vi "Voltage Measurement.vi"() -> ()   [LabVIEW 2021, in "Main.lvlib"]
uses:
  Main.lvlib
  SMU/SMU.lvlib
  DMM/DMM.lvlib
  <instrlib>/niDMM/nidmm.llb/niDMM Resolution in Digits.ctl
  controls/Voltage Config.ctl
  controls/Current Config.ctl
panel:
  out "Current Measurement":dbl
  out "Voltage Measurement":dbl
  in  "Current Config":T1={"Current Limit"=0.01, "Current Limit Range"=0.01} {"Current Limit Range" format="%.3p"; "Current Limit" format="%.3p"}
  in  "Voltage Config":T2={"Voltage Level"=2.0, "Voltage Level Range"=6.0} {"Voltage Level Range" format="%.5p"; "Voltage Level" format="%.5p"}
  out "Signal Out of Range":bool
  out "Measurement":dbl format="%.6p"
  in  "Resolution in Digits":T3=5.5 items=["3 1/2"=3.5, "4 1/2"=4.5, "5 1/2"=5.5, "6 1/2"=6.5, "7 1/2"=7.5]
  in  "Range":dbl=10.0 format="%.2f"
  in  "Device Name":refnum<k15>="Dev1"
  out "error out":errorcluster
  in  "error in":errorcluster
  in  "Vin SMU Channel":string="0"
  in  "Vin SMU":refnum<k15>="Dev1"
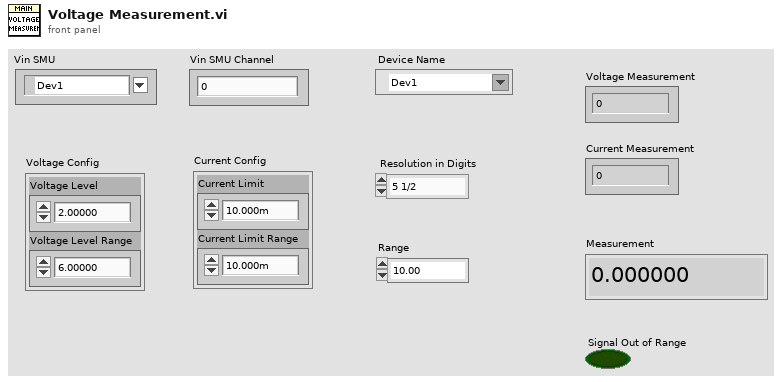
[diagram p1: front panel]
types:
  T1 = typedef "Main.lvlib/Current Config.ctl" = cluster{"Current Limit":dbl, "Current Limit Range":dbl}
  T2 = typedef "Main.lvlib/Voltage Config.ctl" = cluster{"Voltage Level":dbl, "Voltage Level Range":dbl}
  T3 = typedef "niDMM Resolution in Digits.ctl" = dbl
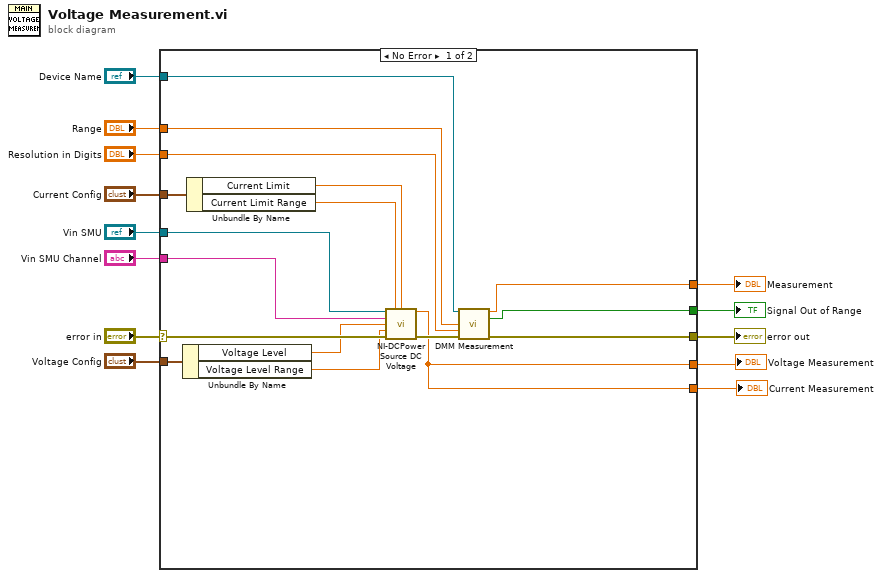
[diagram p0: block diagram]
diagram:
  n1 = case shown="No Error" "error in" {
    selector: "error in" -> [w28 w31]
    tunnel: "Vin SMU" -> [w30 _]
    tunnel: "Vin SMU Channel" -> [w29 _]
    tunnel: [w27 w31] -> w10
    tunnel: "Device Name" -> [w25 _]
    tunnel: "Range" -> [w24 _]
    tunnel: "Resolution in Digits" -> [w23 _]
    tunnel: [w22 _] -> w6
    tunnel: [w21 _] -> w5
    tunnel: "Voltage Config" -> [w20 _]
    tunnel: "Current Config" -> [w17 _]
    tunnel: [w14 _] -> w2
    tunnel: [w14 _] -> w1
    frame No Error {
      n2 = Unbundle By Name(w20) -> ("Voltage Level"=w19:dbl, "Voltage Level Range"=w18:dbl)
      n3 = Unbundle By Name(w17) -> ("Current Limit"=w16:dbl, "Current Limit Range"=w15:dbl)
      n4 = call "NI-DCPower Source DC Voltage.vi"("Vin SMU"=w30, "Current Limit"=w15, "Current Limit Range"=w16, "Vin SMU Channel"=w29, "Voltage Level"=w19, "Voltage Level Range"=w18, "error in"=w28) -> ("Voltage Measurement"=w14:dbl, "error out"=w26:errorcluster)  [unwired: 6 in, 1 out]
      n5 = call "DMM Measurement.vi"("Device Name"=w25, "Range"=w24, "Resolution in Digits"=w23, "error in"=w26) -> ("Measurement"=w22:dbl, "Signal Out of Range"=w21:bool, "error out"=w27:errorcluster)  [unwired: 9 in]
    }
    frame Error {
    }
  }
  "error out" <- w10
  "Measurement" <- w6
  "Signal Out of Range" <- w5
  "Voltage Measurement" <- w2
  "Current Measurement" <- w1
